vi "滤波参数.vi"(11 "x":dbl format="%0.2f") -> (3 "mode":dbl caption="众数" format="%0.2f")   [LabVIEW 2016, in "斯坦道多参数.lvlib"]
uses:
  <vilib>/ptbypt/NI_PtbyPt.lvlib
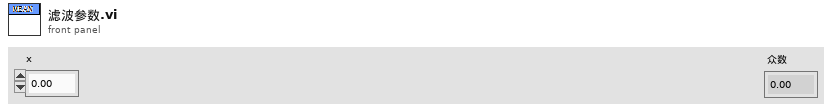
[diagram p1: front panel]
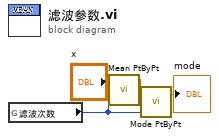
[diagram p0: block diagram]
diagram:
  n1 = global read "断电保存变量.vi" "滤波次数"() -> (w1:u32)
  n2 = call <vilib>:"Mean PtByPt.vi"("x"="x", "sample length"=w1) -> ("mean"=w4:dbl)  [unwired: 2 in, 1 out]
  n3 = call <vilib>:"Mode PtByPt.vi"("sample length"=w1, "x"=w4) -> ("mode"=→"mode":dbl)  [unwired: 2 in, 1 out]
